vi "Convert g & s Arrays to Phasor Array.vi"(7 "s":dbl[](array[numeric]), 9 "g":dbl[](array[numeric])) -> (2 "Phasor Array":T1[](array[typedef]))   [LabVIEW 2019]
uses:
  Phasor (g, s).ctl
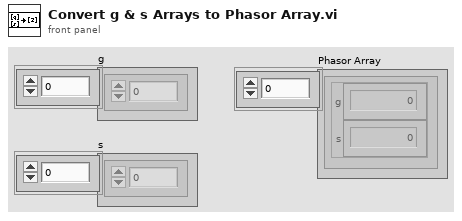
[diagram p1: front panel]
types:
  T1 = typedef "Phasor (g, s).ctl" = cluster{"g":dbl, "s":dbl}
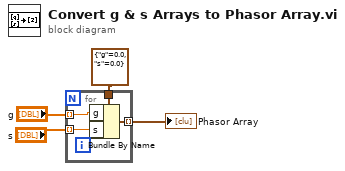
[diagram p0: block diagram]
diagram:
  n1 = for {
    tunnel: "g" -> [w8] mode=indexing
    tunnel: "s" -> [w7] mode=indexing
    tunnel: [w6] -> w2 mode=indexing
    tunnel: T1 {"g"=0.0, "s"=0.0} ("Phasor Array") -> [w5]
    n2 = Bundle By Name(cluster=w5, "g"=w8, "s"=w7) -> (w6:T1)
  }
  "Phasor Array" <- w2
